vi "CircularBuffer.GetElements.vi"(8 "error in (no error)":errorcluster, 11 "CircularBuffer in":refnum<class "CircularBuffer.lvclass">) -> (0 "error out":errorcluster, 2 "Elements":refnum<data-value>[](array[refnum]), 3 "CircularBuffer out":refnum<class "CircularBuffer.lvclass">)   [LabVIEW 2016, in "CircularBuffer.lvclass"]
uses:
  CircularBuffer.lvclass
  types/type/type.lvclass
  CircularBuffer.lvclass/CircularBuffer.ctl
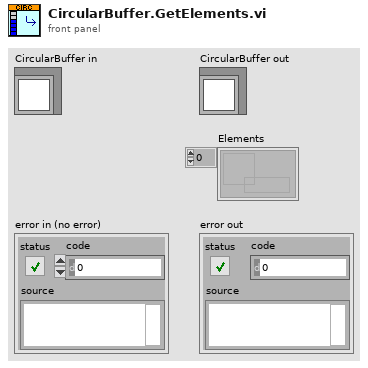
[diagram p1: front panel]
types:
  T1 = typedef "CircularBuffer.lvclass/PrivateData--Ref.ctl" = refnum<data-value>
  T2 = typedef "CircularBuffer.lvclass/PrivateData--Cluster.ctl" = cluster{"Public Events":T3, "Protected Events":T4, "Private Events":T5, "BufferSize":i32, "CurrentElement":i32, "Elements":refnum<data-value>[], "type":refnum<class "type.lvclass">}
  T3 = typedef "CircularBuffer.lvclass/PublicEvents--Cluster.ctl" = cluster{"Buffer Resize Event":refnum<user-event>}
  T4 = typedef "CircularBuffer.lvclass/ProtectedEvents--Cluster.ctl" = cluster{"placeholder":refnum<user-event>}
  T5 = typedef "CircularBuffer.lvclass/PrivateEvents--Cluster.ctl" = cluster{"New Value":refnum<user-event>, "GetElement":refnum<user-event>, "Initialize":refnum<user-event>}
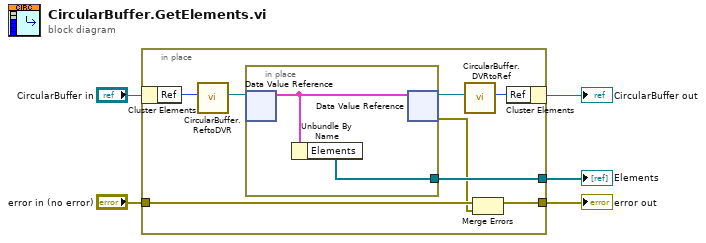
[diagram p0: block diagram]
diagram:
  n1 = in-place {
    in-place-border: [w9] -> w3
    in-place-border: "error in (no error)" -> [w8]
    in-place-border: [w6] -> w5
    n2 = in-place-cluster #1("CircularBuffer in") -> ("Ref"=w13:u32)
    n3 = call "CircularBuffer.ReftoDVR.vi"("Ref"=w13) -> ("Ref"=w11:T1)  [unwired: 10 in]
    n4 = in-place {
      in-place-border: [w15] -> w9
      n5 = in-place-dvr #2(w11) -> (w14:T2)  [unwired: 1 out]
      n6 = Unbundle By Name(w14) -> ("Elements"=w15:refnum<data-value>[])
      n7 = in-place-dvr #2(w14) -> (w10:T1, w7:errorcluster)
    }
    n8 = call "CircularBuffer.DVRtoRef.vi"("Ref"=w10) -> ("Ref"=w12:u32)  [unwired: 10 in]
    n9 = Merge Errors(w8, w7) -> (w6:errorcluster)
    n10 = in-place-cluster #1("Ref"=w12) -> (→"CircularBuffer out":refnum<class "CircularBuffer.lvclass">)
  }
  "error out" <- w5
  "Elements" <- w3
